vi "MARS_RESET.vi"(8 "error in":errorcluster, 11 "VISA Resource":refnum<visa-resource-name>) -> (0 "error out":errorcluster, 3 "VISA resource name out":refnum<visa-resource-name>)   [LabVIEW 2015]
uses:
  MARS_Global_var.vi
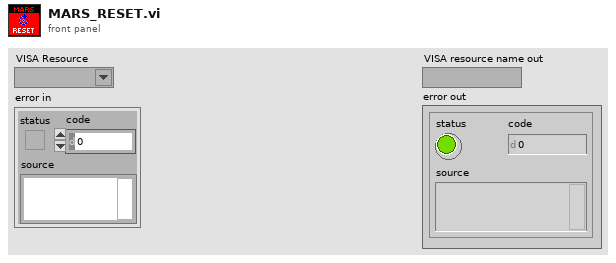
[diagram p1: front panel]
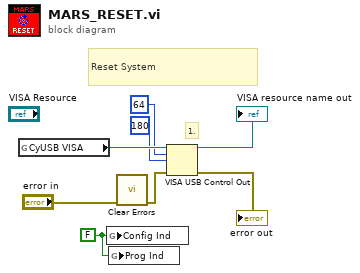
[diagram p0: block diagram]
diagram:
  w8 = FALSE ("Config Ind")
  # "Reset System"
  # "1."
  n1 = global read "MARS_Global_var.vi" "CyUSB VISA"() -> (w5:refnum<visa-resource-name>)
  n2 = global write "MARS_Global_var.vi" "Config Ind"(w8) -> ()
  n3 = global write "MARS_Global_var.vi" "Prog Ind"(w8) -> ()
  n4 = call <vilib>:"Clear Errors.vi"("error in (no error)"="error in") -> ("error out"=w2:errorcluster)  [unwired: 5 in, 1 out]
  n5 = VISA USB Control Out(0:w5, 5:i16 64 ("request type"), 7:i16 180 ("request type"), 11:w2) -> (4:→"VISA resource name out":refnum<visa-resource-name>, 15:→"error out":errorcluster)  [unwired: 3 in]
